vi "Sequence Module.vi"(0 "control_request":string, 5 "control_sequence_file_path":path, 9 "control_sequence_parameters":T3, 11 "control_sequence_current_parameters":T1) -> (3 "indicator_sequence_current_parameters":T1, 4 "indicator_sequence_parameters":T2, 6 "indicator_sequence_move_x":bool, 8 "indicator_UV_activation_intensity":dbl, 10 "indicator_sequence_move_y":bool, 13 "indicator_sequence_distance_y":dbl, 14 "indicator_UV_activation_time":dbl, 15 "indicator_sequence_distance_x":dbl)   [LabVIEW 2020]
uses:
  <vilib>/Utility/file.llb/Read Delimited Spreadsheet (string).vi
panel:
  out "indicator_saved_positions":i64[][](array[numeric])
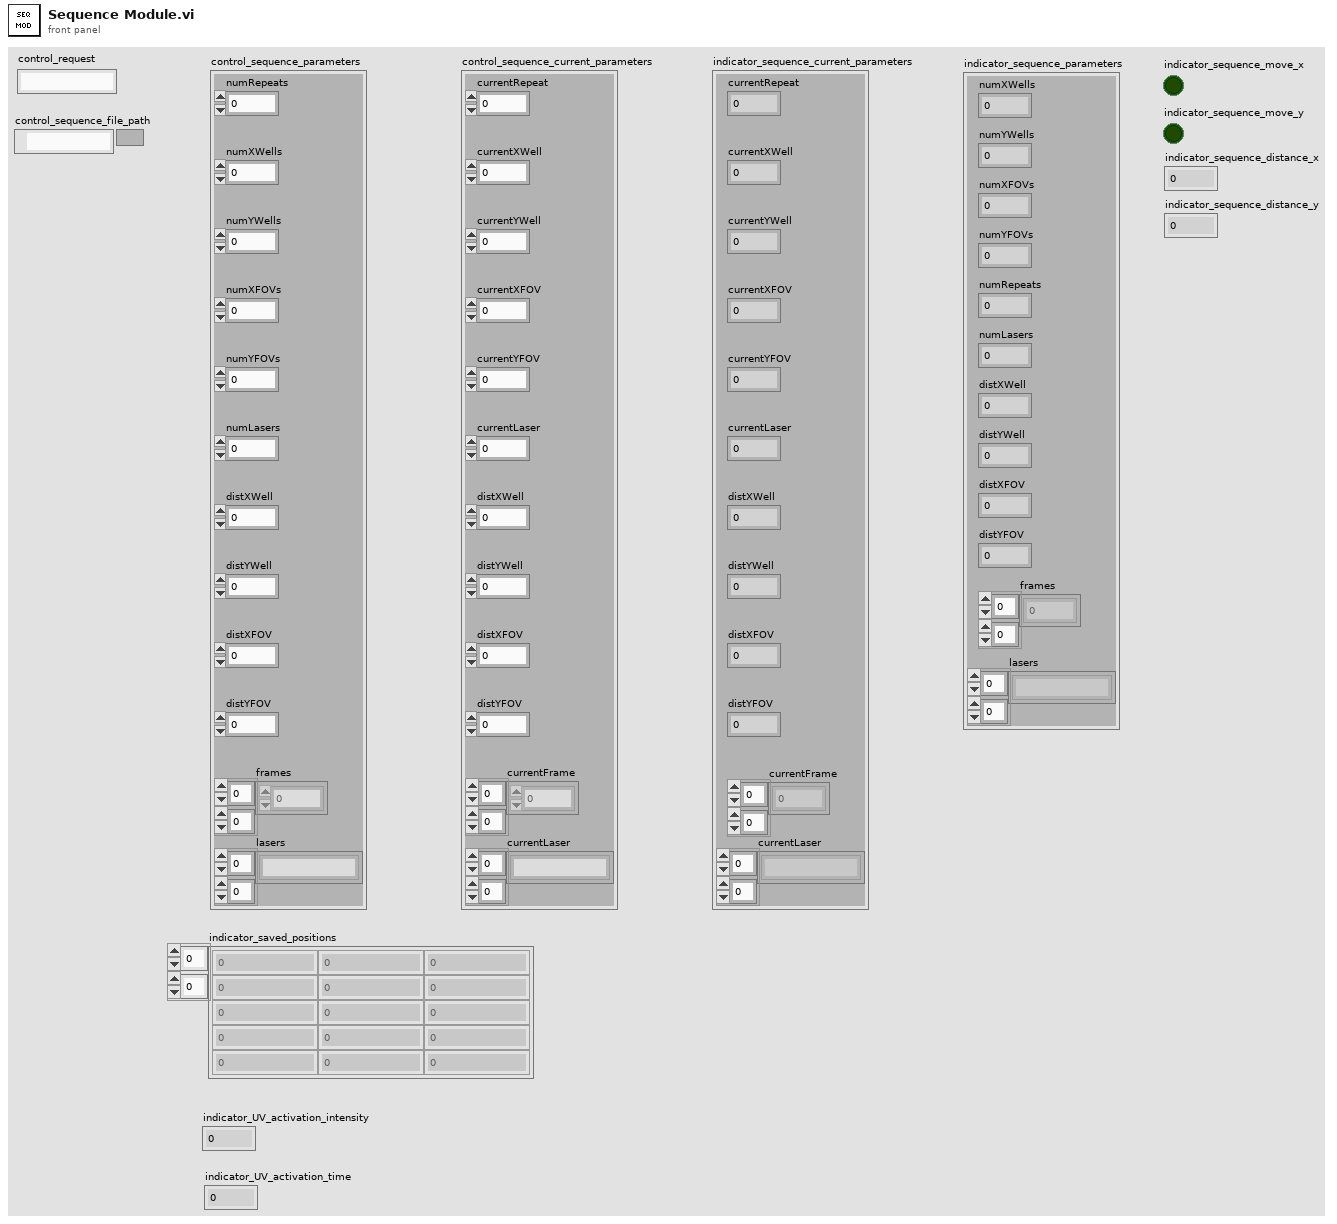
[diagram p1: front panel]
types:
  T1 = cluster{"currentXWell":i32, "currentYWell":i32, "currentXFOV":i32, "currentYFOV":i32, "currentRepeat":i32, "currentLaser":i32, "distXWell":i32, "distYWell":i32, "distXFOV":i32, "distYFOV":i32, "currentFrame":i32[][], "currentLaser":string[][]}
  T2 = cluster{"numXWells":i32, "numYWells":i32, "numXFOVs":i32, "numYFOVs":i32, "numRepeats":i32, "numLasers":i32, "distXWell":i32, "distYWell":i32, "distXFOV":i32, "distYFOV":i32, "frames":i32[][], "lasers":string[][]}
  T3 = cluster{"numXWells":i32, "numYWells":i32, "numXFOVs":i32, "numYFOVs":i32, "numRepeats":i32, "numLasers":i32, "distXWell":i32, "distYWell":i32, "distXFOV":i32, "distYFOV":i32, "frames":u32[][], "lasers":string[][]}
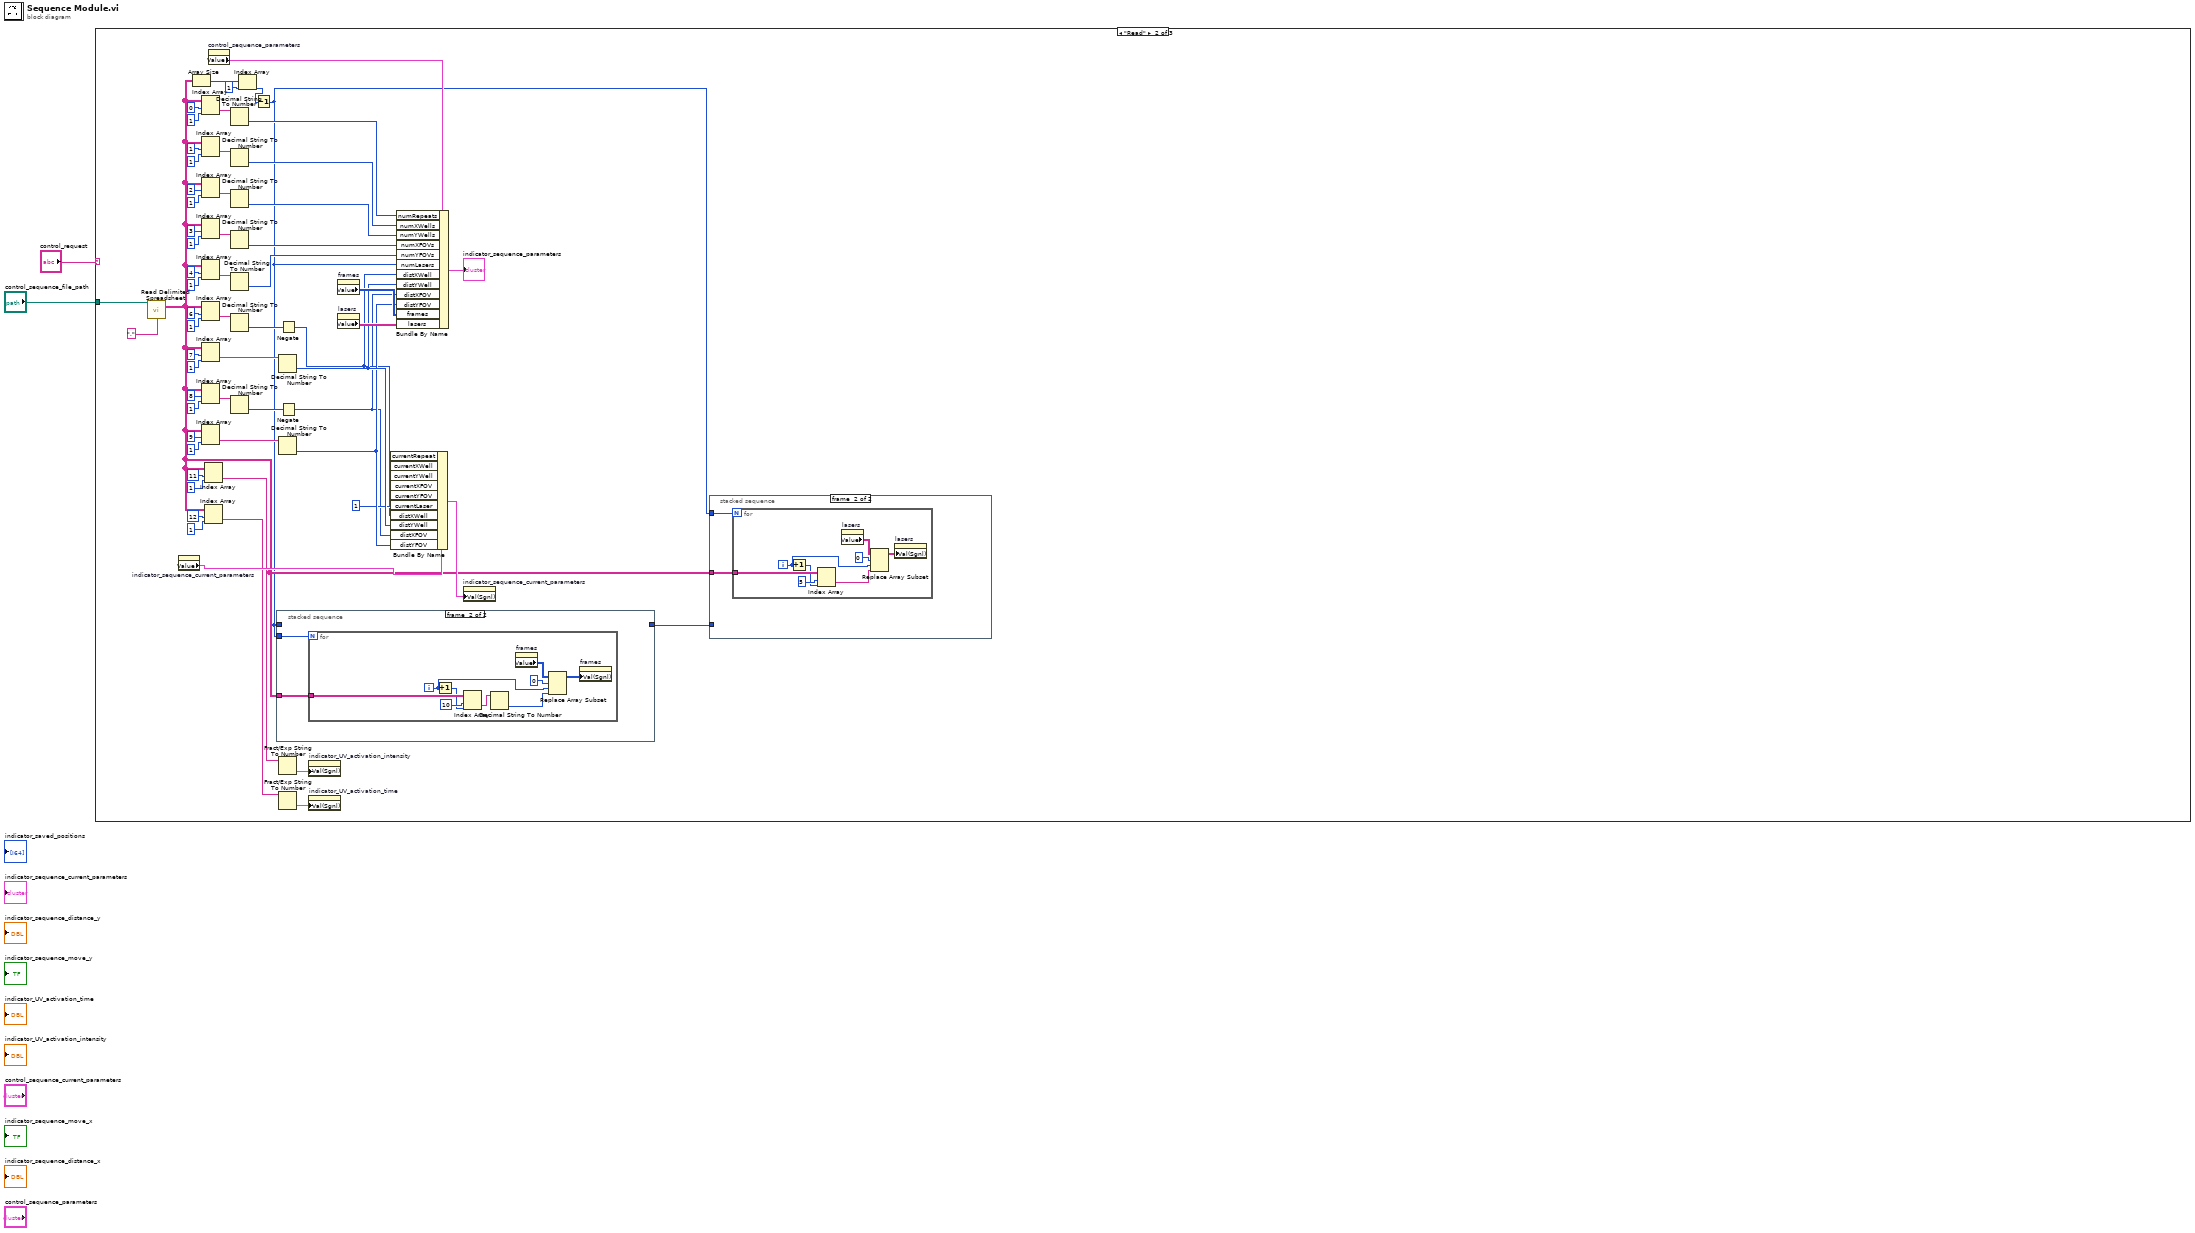
[diagram p0: block diagram]
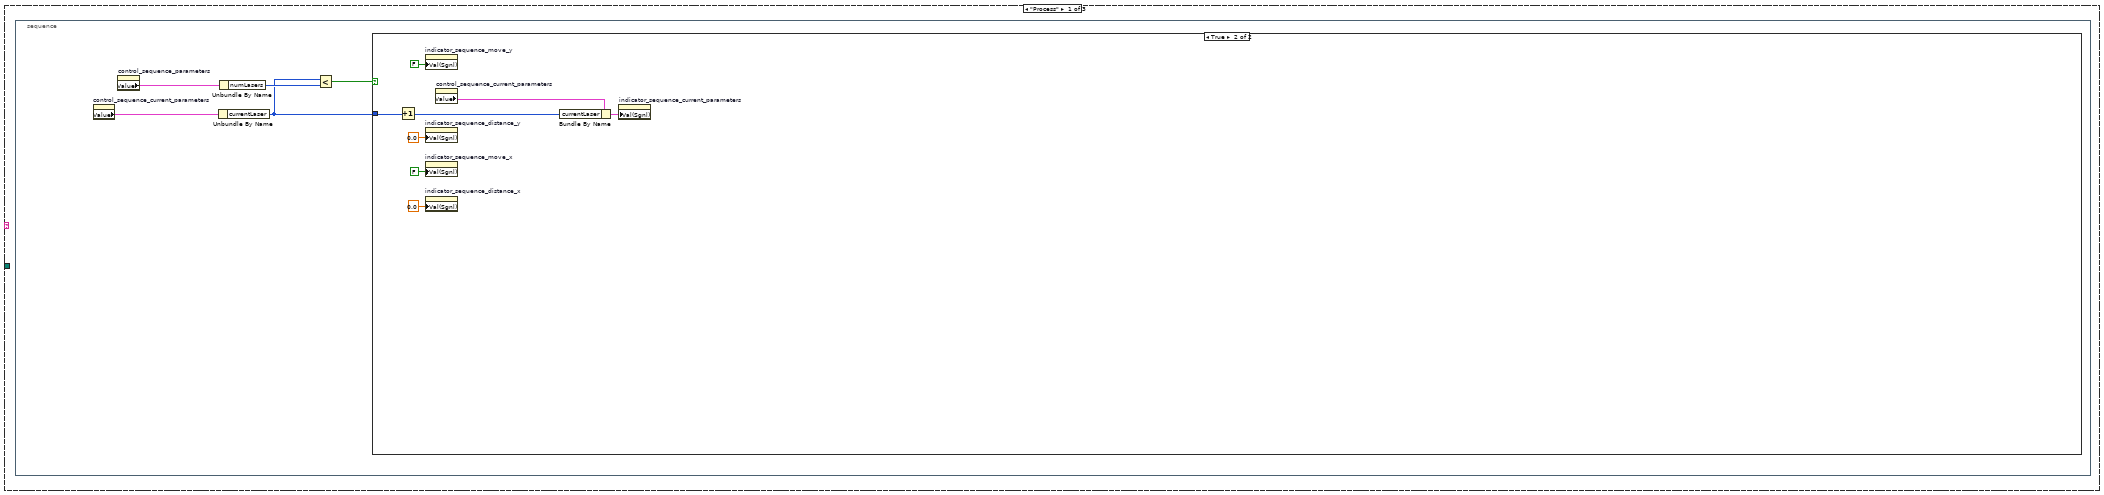
[diagram p2: hidden frame]
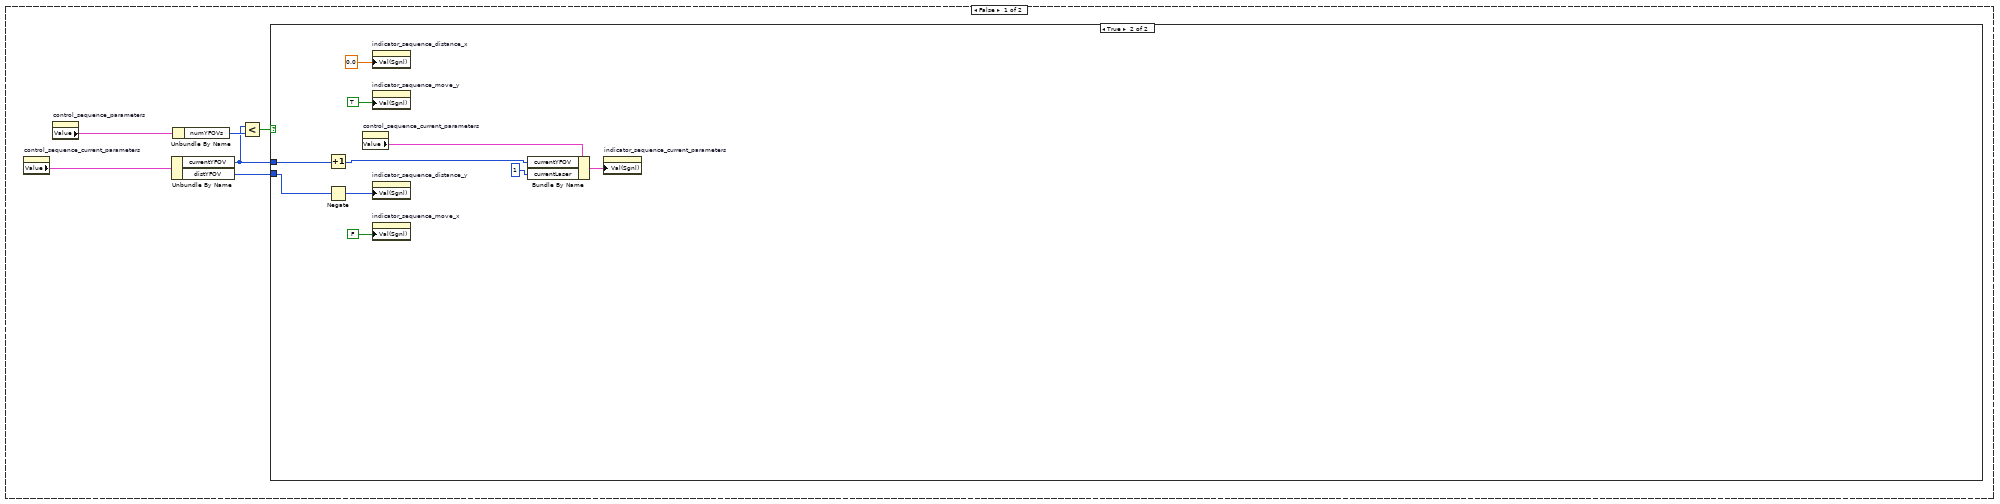
[diagram p3: hidden frame]
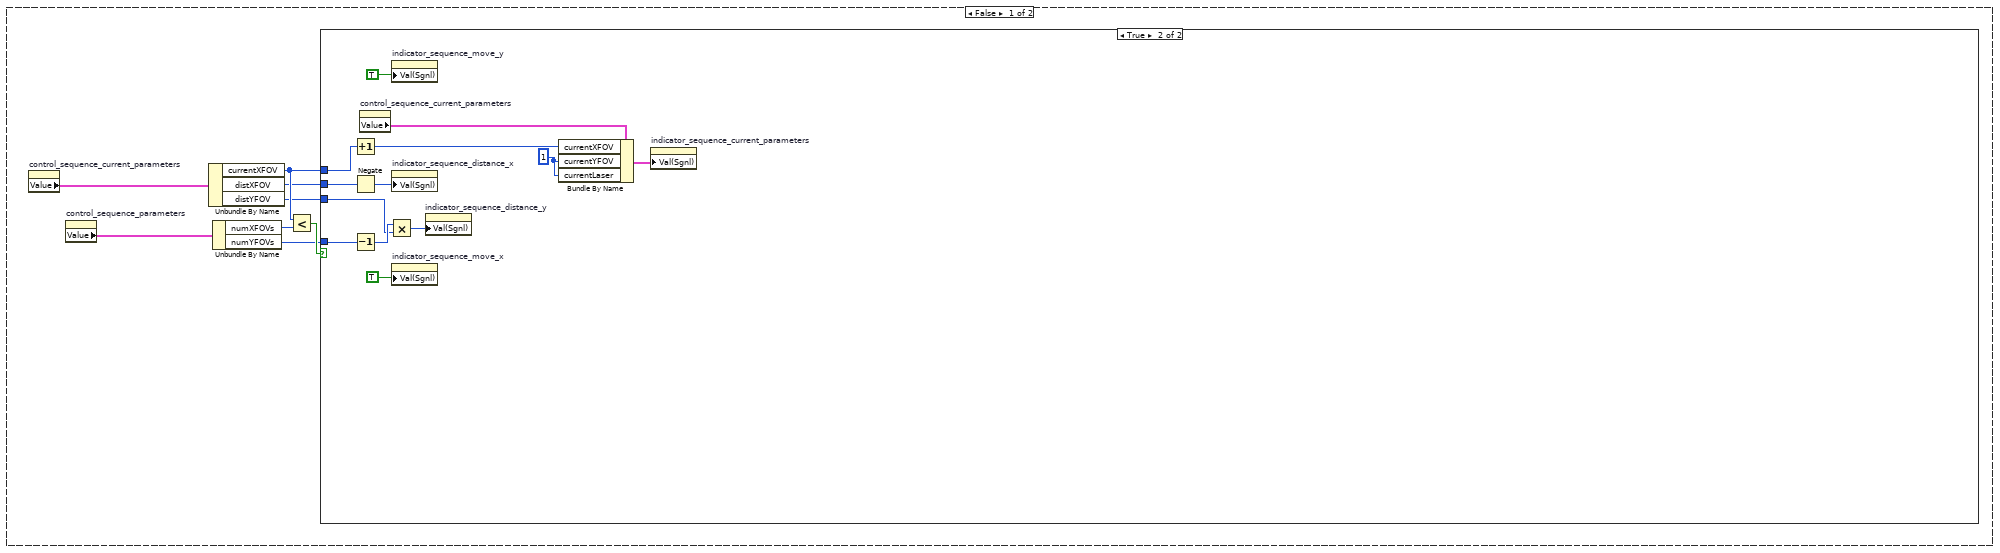
[diagram p4: hidden frame]
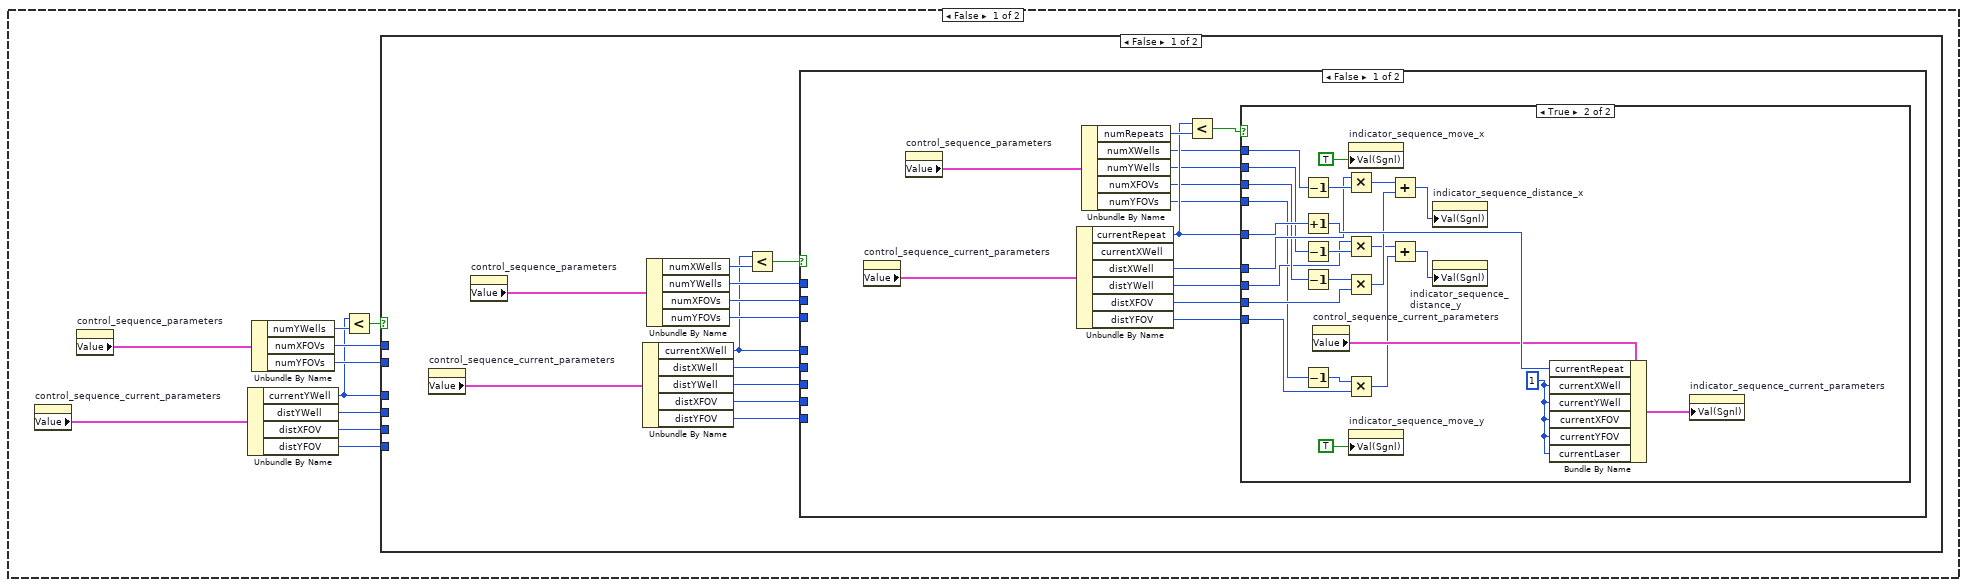
[diagram p5: hidden frame]
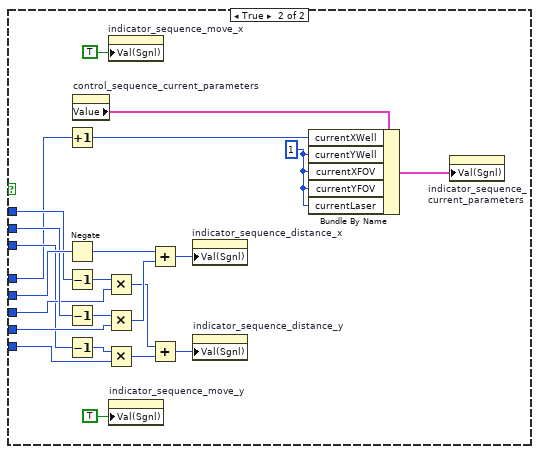
[diagram p7: hidden frame]
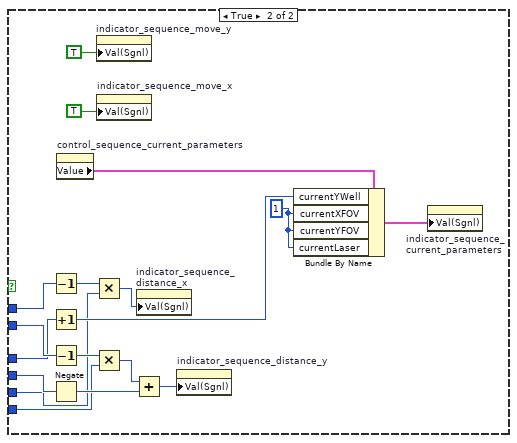
[diagram p8: hidden frame]
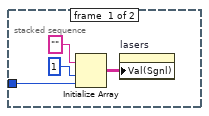
[diagram p9: hidden frame]
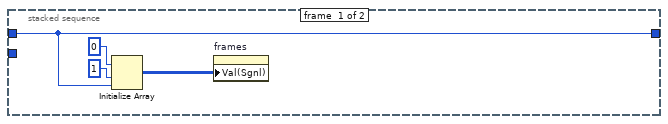
[diagram p10: hidden frame]
diagram:
  n1 = case shown="\"Read\"" "control_request" {
    tunnel: "control_sequence_file_path" -> [_ w171 _]
    frame "Process" {
      n2 = stacked-sequence {
        frame #0 {
          n3 = property on="control_sequence_current_parameters" class="Clust (strict)"() -> ("Value"=w6:T1)  [unwired: 2 in, 2 out]
          n4 = property on="control_sequence_parameters" class="Clust (strict)"() -> ("Value"=w5:T3)  [unwired: 2 in, 2 out]
          n5 = Unbundle By Name(w6) -> ("currentLaser"=w3:i32)
          n6 = Unbundle By Name(w5) -> ("numLasers"=w4:i32)
          n7 = Less?(x=w3, y=w4) -> (x < y?=w7:bool)
          n8 = case shown="True" w7 {
            tunnel: w3 -> [_ w146]
            frame False {
              n9 = property on="control_sequence_current_parameters" class="Clust (strict)"() -> ("Value"=w12:T1)  [unwired: 2 in, 2 out]
              n10 = property on="control_sequence_parameters" class="Clust (strict)"() -> ("Value"=w11:T3)  [unwired: 2 in, 2 out]
              n11 = Unbundle By Name(w12) -> ("currentYFOV"=w8:i32, "distYFOV"=w9:i32)
              n12 = Unbundle By Name(w11) -> ("numYFOVs"=w10:i32)
              n13 = Less?(x=w8, y=w10) -> (x < y?=w13:bool)
              n14 = case shown="True" w13 {
                tunnel: w9 -> [_ w137]
                tunnel: w8 -> [_ w136]
                frame False {
                  n15 = property on="control_sequence_current_parameters" class="Clust (strict)"() -> ("Value"=w20:T1)  [unwired: 2 in, 2 out]
                  n16 = property on="control_sequence_parameters" class="Clust (strict)"() -> ("Value"=w19:T3)  [unwired: 2 in, 2 out]
                  n17 = Unbundle By Name(w20) -> ("currentXFOV"=w17:i32, "distXFOV"=w16:i32, "distYFOV"=w14:i32)
                  n18 = Unbundle By Name(w19) -> ("numXFOVs"=w18:i32, "numYFOVs"=w15:i32)
                  n19 = Less?(x=w17, y=w18) -> (x < y?=w21:bool)
                  n20 = case shown="True" w21 {
                    tunnel: w17 -> [_ w126]
                    tunnel: w16 -> [_ w125]
                    tunnel: w15 -> [_ w124]
                    tunnel: w14 -> [_ w123]
                    frame False {
                      n21 = property on="control_sequence_current_parameters" class="Clust (strict)"() -> ("Value"=w30:T1)  [unwired: 2 in, 2 out]
                      n22 = property on="control_sequence_parameters" class="Clust (strict)"() -> ("Value"=w29:T3)  [unwired: 2 in, 2 out]
                      n23 = Unbundle By Name(w30) -> ("currentYWell"=w22:i32, "distYWell"=w27:i32, "distXFOV"=w23:i32, "distYFOV"=w25:i32)
                      n24 = Unbundle By Name(w29) -> ("numYWells"=w28:i32, "numXFOVs"=w24:i32, "numYFOVs"=w26:i32)
                      n25 = Less?(x=w22, y=w28) -> (x < y?=w31:bool)
                      n26 = case shown="False" w31 {
                        tunnel: w27 -> [_ w110]
                        tunnel: w26 -> [_ w109]
                        tunnel: w25 -> [_ w108]
                        tunnel: w24 -> [_ w107]
                        tunnel: w23 -> [_ w106]
                        tunnel: w22 -> [_ w105]
                        frame False {
                          n27 = property on="control_sequence_current_parameters" class="Clust (strict)"() -> ("Value"=w42:T1)  [unwired: 2 in, 2 out]
                          n28 = property on="control_sequence_parameters" class="Clust (strict)"() -> ("Value"=w41:T3)  [unwired: 2 in, 2 out]
                          n29 = Unbundle By Name(w42) -> ("currentXWell"=w32:i32, "distXWell"=w39:i32, "distYWell"=w35:i32, "distXFOV"=w37:i32, "distYFOV"=w33:i32)
                          n30 = Unbundle By Name(w41) -> ("numXWells"=w40:i32, "numYWells"=w36:i32, "numXFOVs"=w38:i32, "numYFOVs"=w34:i32)
                          n31 = Less?(x=w32, y=w40) -> (x < y?=w43:bool)
                          n32 = case shown="False" w43 {
                            tunnel: w39 -> [_ w89]
                            tunnel: w38 -> [_ w88]
                            tunnel: w37 -> [_ w87]
                            tunnel: w36 -> [_ w86]
                            tunnel: w35 -> [_ w85]
                            tunnel: w34 -> [_ w84]
                            tunnel: w33 -> [_ w83]
                            tunnel: w32 -> [_ w82]
                            frame False {
                              n33 = property on="control_sequence_current_parameters" class="Clust (strict)"() -> ("Value"=w55:T1)  [unwired: 2 in, 2 out]
                              n34 = property on="control_sequence_parameters" class="Clust (strict)"() -> ("Value"=w54:T3)  [unwired: 2 in, 2 out]
                              n35 = Unbundle By Name(w55) -> ("currentRepeat"=w52:i32, "distXWell"=w50:i32, "distYWell"=w47:i32, "distXFOV"=w48:i32, "distYFOV"=w45:i32)  [unwired: 1 out]
                              n36 = Unbundle By Name(w54) -> ("numRepeats"=w53:i32, "numXWells"=w51:i32, "numYWells"=w46:i32, "numXFOVs"=w49:i32, "numYFOVs"=w44:i32)
                              n37 = Less?(x=w52, y=w53) -> (x < y?=w56:bool)
                              n38 = case shown="True" w56 {
                                tunnel: w52 -> [_ w75]
                                tunnel: w51 -> [_ w74]
                                tunnel: w50 -> [_ w72]
                                tunnel: w49 -> [_ w68]
                                tunnel: w48 -> [_ w67]
                                tunnel: w47 -> [_ w60]
                                tunnel: w46 -> [_ w59]
                                tunnel: w45 -> [_ w58]
                                tunnel: w44 -> [_ w57]
                                frame False {
                                }
                                frame True {
                                w78 = 1 ("currentXWell")
                                n39 = Decrement(x=w74) -> (x-1=w73:i32)
                                n40 = Increment(x=w75) -> (x+1=w80:i32)
                                n41 = Decrement(x=w59) -> (x-1=w65:i32)
                                n42 = Decrement(x=w68) -> (x-1=w69:i32)
                                n43 = Decrement(x=w57) -> (x-1=w62:i32)
                                n44 = property on="control_sequence_current_parameters" class="Clust (strict)"() -> ("Value"=w79:T1)  [unwired: 2 in, 2 out]
                                n45 = Multiply(x=w72, y=w73) -> (x*y=w71:i32)
                                n46 = Multiply(x=w60, y=w65) -> (x*y=w64:i32)
                                n47 = Multiply(x=w69, y=w67) -> (x*y=w70:i32)
                                n48 = Multiply(x=w62, y=w58) -> (x*y=w63:i32)
                                n49 = property on="indicator_sequence_move_x" class="Bool (strict)"("Val(Sgnl)"=TRUE ("Value (Signaling)")) -> ()  [unwired: 2 in, 2 out]
                                n50 = property on="indicator_sequence_move_y" class="Bool (strict)"("Val(Sgnl)"=TRUE ("Value (Signaling)")) -> ()  [unwired: 2 in, 2 out]
                                n51 = Add(x=w71, y=w70) -> (x+y=w66:i32)
                                n52 = Add(x=w64, y=w63) -> (x+y=w61:i32)
                                n53 = property on="indicator_sequence_distance_x" class="DigNum (strict)"("Val(Sgnl)"=w66) -> ()  [unwired: 2 in, 2 out]
                                n54 = property on="indicator_sequence_distance_y" class="DigNum (strict)"("Val(Sgnl)"=w61) -> ()  [unwired: 2 in, 2 out]
                                n55 = Bundle By Name(cluster=w79, "currentRepeat"=w80, "currentXWell"=w78, "currentYWell"=w78, "currentXFOV"=w78, "currentYFOV"=w78, "currentLaser"=w78) -> (w81:T1)
                                n56 = property on="indicator_sequence_current_parameters" class="Clust (strict)"("Val(Sgnl)"=w81) -> ()  [unwired: 2 in, 2 out]
                                }
                              }
                            }
                            frame True {
                              w101 = 1 ("currentYWell")
                              n57 = Increment(x=w82) -> (x+1=w103:i32)
                              n58 = Negate(x=w89) -> (-x=w95:i32)
                              n59 = Decrement(x=w86) -> (x-1=w98:i32)
                              n60 = Decrement(x=w88) -> (x-1=w97:i32)
                              n61 = Decrement(x=w84) -> (x-1=w96:i32)
                              n62 = property on="control_sequence_current_parameters" class="Clust (strict)"() -> ("Value"=w102:T1)  [unwired: 2 in, 2 out]
                              n63 = Multiply(x=w98, y=w85) -> (x*y=w92:i32)
                              n64 = Multiply(x=w97, y=w87) -> (x*y=w94:i32)
                              n65 = Multiply(x=w96, y=w83) -> (x*y=w91:i32)
                              n66 = property on="indicator_sequence_move_x" class="Bool (strict)"("Val(Sgnl)"=TRUE ("Value (Signaling)")) -> ()  [unwired: 2 in, 2 out]
                              n67 = property on="indicator_sequence_move_y" class="Bool (strict)"("Val(Sgnl)"=TRUE ("Value (Signaling)")) -> ()  [unwired: 2 in, 2 out]
                              n68 = Add(x=w95, y=w94) -> (x+y=w93:i32)
                              n69 = Add(x=w92, y=w91) -> (x+y=w90:i32)
                              n70 = property on="indicator_sequence_distance_x" class="DigNum (strict)"("Val(Sgnl)"=w93) -> ()  [unwired: 2 in, 2 out]
                              n71 = property on="indicator_sequence_distance_y" class="DigNum (strict)"("Val(Sgnl)"=w90) -> ()  [unwired: 2 in, 2 out]
                              n72 = Bundle By Name(cluster=w102, "currentXWell"=w103, "currentYWell"=w101, "currentXFOV"=w101, "currentYFOV"=w101, "currentLaser"=w101) -> (w104:T1)
                              n73 = property on="indicator_sequence_current_parameters" class="Clust (strict)"("Val(Sgnl)"=w104) -> ()  [unwired: 2 in, 2 out]
                            }
                          }
                        }
                        frame True {
                          w119 = 1 ("currentXFOV")
                          n74 = Decrement(x=w107) -> (x-1=w116:i32)
                          n75 = Increment(x=w105) -> (x+1=w121:i32)
                          n76 = Decrement(x=w109) -> (x-1=w114:i32)
                          n77 = Negate(x=w110) -> (-x=w113:i32)
                          n78 = property on="control_sequence_current_parameters" class="Clust (strict)"() -> ("Value"=w120:T1)  [unwired: 2 in, 2 out]
                          n79 = Multiply(x=w116, y=w106) -> (x*y=w115:i32)
                          n80 = Multiply(x=w114, y=w108) -> (x*y=w112:i32)
                          n81 = property on="indicator_sequence_move_y" class="Bool (strict)"("Val(Sgnl)"=TRUE ("Value (Signaling)")) -> ()  [unwired: 2 in, 2 out]
                          n82 = property on="indicator_sequence_move_x" class="Bool (strict)"("Val(Sgnl)"=TRUE ("Value (Signaling)")) -> ()  [unwired: 2 in, 2 out]
                          n83 = Add(x=w112, y=w113) -> (x+y=w111:i32)
                          n84 = property on="indicator_sequence_distance_x" class="DigNum (strict)"("Val(Sgnl)"=w115) -> ()  [unwired: 2 in, 2 out]
                          n85 = property on="indicator_sequence_distance_y" class="DigNum (strict)"("Val(Sgnl)"=w111) -> ()  [unwired: 2 in, 2 out]
                          n86 = Bundle By Name(cluster=w120, "currentYWell"=w121, "currentXFOV"=w119, "currentYFOV"=w119, "currentLaser"=w119) -> (w122:T1)
                          n87 = property on="indicator_sequence_current_parameters" class="Clust (strict)"("Val(Sgnl)"=w122) -> ()  [unwired: 2 in, 2 out]
                        }
                      }
                    }
                    frame True {
                      w132 = 1 ("currentYFOV")
                      n88 = Increment(x=w126) -> (x+1=w135:i32)
                      n89 = Negate(x=w125) -> (-x=w129:i32)
                      n90 = Decrement(x=w124) -> (x-1=w128:i32)
                      n91 = property on="control_sequence_current_parameters" class="Clust (strict)"() -> ("Value"=w133:T1)  [unwired: 2 in, 2 out]
                      n92 = Multiply(x=w128, y=w123) -> (x*y=w127:i32)
                      n93 = property on="indicator_sequence_move_y" class="Bool (strict)"("Val(Sgnl)"=TRUE ("Value (Signaling)")) -> ()  [unwired: 2 in, 2 out]
                      n94 = property on="indicator_sequence_distance_x" class="DigNum (strict)"("Val(Sgnl)"=w129) -> ()  [unwired: 2 in, 2 out]
                      n95 = property on="indicator_sequence_move_x" class="Bool (strict)"("Val(Sgnl)"=TRUE ("Value (Signaling)")) -> ()  [unwired: 2 in, 2 out]
                      n96 = property on="indicator_sequence_distance_y" class="DigNum (strict)"("Val(Sgnl)"=w127) -> ()  [unwired: 2 in, 2 out]
                      n97 = Bundle By Name(cluster=w133, "currentXFOV"=w135, "currentYFOV"=w132, "currentLaser"=w132) -> (w134:T1)
                      n98 = property on="indicator_sequence_current_parameters" class="Clust (strict)"("Val(Sgnl)"=w134) -> ()  [unwired: 2 in, 2 out]
                    }
                  }
                }
                frame True {
                  n99 = Increment(x=w136) -> (x+1=w143:i32)
                  n100 = Negate(x=w137) -> (-x=w139:i32)
                  n101 = property on="control_sequence_current_parameters" class="Clust (strict)"() -> ("Value"=w144:T1)  [unwired: 2 in, 2 out]
                  n102 = property on="indicator_sequence_distance_x" class="DigNum (strict)"("Val(Sgnl)"=0.0 ("Value (Signaling)")) -> ()  [unwired: 2 in, 2 out]
                  n103 = property on="indicator_sequence_move_y" class="Bool (strict)"("Val(Sgnl)"=TRUE ("Value (Signaling)")) -> ()  [unwired: 2 in, 2 out]
                  n104 = property on="indicator_sequence_distance_y" class="DigNum (strict)"("Val(Sgnl)"=w139) -> ()  [unwired: 2 in, 2 out]
                  n105 = property on="indicator_sequence_move_x" class="Bool (strict)"("Val(Sgnl)"=FALSE ("Value (Signaling)")) -> ()  [unwired: 2 in, 2 out]
                  n106 = Bundle By Name(cluster=w144, "currentYFOV"=w143, "currentLaser"=1) -> (w145:T1)
                  n107 = property on="indicator_sequence_current_parameters" class="Clust (strict)"("Val(Sgnl)"=w145) -> ()  [unwired: 2 in, 2 out]
                }
              }
            }
            frame True {
              n108 = Increment(x=w146) -> (x+1=w153:i32)
              n109 = property on="indicator_sequence_move_y" class="Bool (strict)"("Val(Sgnl)"=FALSE ("Value (Signaling)")) -> ()  [unwired: 2 in, 2 out]
              n110 = property on="indicator_sequence_distance_y" class="DigNum (strict)"("Val(Sgnl)"=0.0 ("Value (Signaling)")) -> ()  [unwired: 2 in, 2 out]
              n111 = property on="indicator_sequence_move_x" class="Bool (strict)"("Val(Sgnl)"=FALSE ("Value (Signaling)")) -> ()  [unwired: 2 in, 2 out]
              n112 = property on="indicator_sequence_distance_x" class="DigNum (strict)"("Val(Sgnl)"=0.0 ("Value (Signaling)")) -> ()  [unwired: 2 in, 2 out]
              n113 = property on="control_sequence_current_parameters" class="Clust (strict)"() -> ("Value"=w151:T1)  [unwired: 2 in, 2 out]
              n114 = Bundle By Name(cluster=w151, "currentLaser"=w153) -> (w152:T1)
              n115 = property on="indicator_sequence_current_parameters" class="Clust (strict)"("Val(Sgnl)"=w152) -> ()  [unwired: 2 in, 2 out]
            }
          }
        }
      }
    }
    frame "Read" {
      w170 = 1 ("currentLaser")
      n116 = call-poly <vilib>:"Read Delimited Spreadsheet.vi"("file path (dialog if empty)"=w171, "delimiter (\\t)"="," ("delimiter (\\t)")) -> ("all rows"=w157:string[][])  [unwired: 8 in, 5 out]
      n117 = property on="indicator_sequence_current_parameters" class="Clust (strict)"() -> ("Value"=w179:T1)  [unwired: 2 in, 2 out]
      n118 = Array Size(array=w157) -> (size(s)=w189:i32[])
      n119 = Index Array(array=w157, index (row)=0 ("index"), index (col)=1 ("disabled index (col)")) -> (element=w195:string)
      n120 = Index Array(array=w157, index (row)=1 ("index"), index (col)=1 ("disabled index (col)")) -> (element=w194:string)
      n121 = Index Array(array=w157, index (row)=2 ("index"), index (col)=1 ("disabled index (col)")) -> (element=w193:string)
      n122 = Index Array(array=w157, index (row)=3 ("index"), index (col)=1 ("disabled index (col)")) -> (element=w192:string)
      n123 = Index Array(array=w157, index (row)=4 ("index"), index (col)=1 ("disabled index (col)")) -> (element=w191:string)
      n124 = Index Array(array=w157, index (row)=6 ("index"), index (col)=1 ("disabled index (col)")) -> (element=w188:string)
      n125 = Index Array(array=w157, index (row)=7 ("index"), index (col)=1 ("disabled index (col)")) -> (element=w187:string)
      n126 = Index Array(array=w157, index (row)=8 ("index"), index (col)=1 ("disabled index (col)")) -> (element=w186:string)
      n127 = Index Array(array=w157, index (row)=9 ("index"), index (col)=1 ("disabled index (col)")) -> (element=w185:string)
      n128 = Index Array(array=w157, index (row)=11, index (col)=1 ("disabled index (col)")) -> (element=w162:string)
      n129 = Index Array(array=w157, index (row)=12, index (col)=1 ("disabled index (col)")) -> (element=w158:string)
      n130 = property on="control_sequence_parameters" class="Clust (strict)"() -> ("Value"=w169:T3)  [unwired: 2 in, 2 out]
      n131 = Decimal String To Number(string=w195) -> (number=w178:i32)  [unwired: 2 in, 1 out]
      n132 = Decimal String To Number(string=w194) -> (number=w177:i32)  [unwired: 2 in, 1 out]
      n133 = Decimal String To Number(string=w193) -> (number=w176:i32)  [unwired: 2 in, 1 out]
      n134 = Decimal String To Number(string=w192) -> (number=w175:i32)  [unwired: 2 in, 1 out]
      n135 = Decimal String To Number(string=w191) -> (number=w174:i32)  [unwired: 2 in, 1 out]
      n136 = Decimal String To Number(string=w188) -> (number=w168:i32)  [unwired: 2 in, 1 out]
      n137 = Decimal String To Number(string=w186) -> (number=w166:i32)  [unwired: 2 in, 1 out]
      n138 = Index Array(array=w189, index=1) -> (element=w155:i32)
      n139 = Decrement(x=w155) -> (x-1=w154:i32)
      n140 = stacked-sequence {
        tunnel: w154 -> [w230 _]
        tunnel: [w230 _] -> w184
        tunnel: w154 -> [_ w234]
        tunnel: w157 -> [_ w233]
        frame #0 {
          n141 = Initialize Array(0 ("element"), 1 ("dimension size"), w230) -> (w229:i32[][])
          n142 = property on="frames" class="Arr (strict)"("Val(Sgnl)"=w229) -> ()  [unwired: 2 in, 2 out]
        }
        frame #1 {
          n143 = for {
            N: w234 -> [_]
            tunnel: w233 -> [w243]
            i -> [w235]
            n144 = Increment(x=w235) -> (x+1=w236:i32)
            n145 = Index Array(array=w243, index (row)=10 ("index"), index (col)=w236) -> (element=w241:string)
            n146 = Decimal String To Number(string=w241) -> (number=w239:i32)  [unwired: 2 in, 1 out]
            n147 = property on="frames" class="Arr (strict)"() -> ("Value"=w237:i32[][])  [unwired: 2 in, 2 out]
            n148 = Replace Array Subset(array=w237, new element=w239, index (row)=0, index (col)=w235) -> (w238:i32[][])
            n149 = property on="frames" class="Arr (strict)"("Val(Sgnl)"=w238) -> ()  [unwired: 2 in, 2 out]
          }
        }
      }
      n150 = Decimal String To Number(string=w187) -> (number=w173:i32)  [unwired: 2 in, 1 out]
      n151 = Decimal String To Number(string=w185) -> (number=w172:i32)  [unwired: 2 in, 1 out]
      n152 = Fract/Exp String To Number(string=w162) -> (number=w161:dbl)  [unwired: 3 in, 1 out]
      n153 = Fract/Exp String To Number(string=w158) -> (number=w156:dbl)  [unwired: 3 in, 1 out]
      n154 = Negate(x=w168) -> (-x=w167:i32)
      n155 = Negate(x=w166) -> (-x=w165:i32)
      n156 = property on="indicator_UV_activation_intensity" class="DigNum (strict)"("Val(Sgnl)"=w161) -> ()  [unwired: 2 in, 2 out]
      n157 = property on="indicator_UV_activation_time" class="DigNum (strict)"("Val(Sgnl)"=w156) -> ()  [unwired: 2 in, 2 out]
      n158 = property on="frames" class="Arr (strict)"() -> ("Value"=w182:i32[][])  [unwired: 2 in, 2 out]
      n159 = property on="lasers" class="Arr (strict)"() -> ("Value"=w181:string[][])  [unwired: 2 in, 2 out]
      n160 = Bundle By Name(cluster=w179, "currentRepeat"=w170, "currentXWell"=w170, "currentYWell"=w170, "currentXFOV"=w170, "currentYFOV"=w170, "currentLaser"=w170, "distXWell"=w167, "distYWell"=w173, "distXFOV"=w165, "distYFOV"=w172) -> (w180:T1)
      n161 = Bundle By Name(cluster=w169, "numRepeats"=w178, "numXWells"=w177, "numYWells"=w176, "numXFOVs"=w175, "numYFOVs"=w174, "numLasers"=w154, "distXWell"=w167, "distYWell"=w173, "distXFOV"=w165, "distYFOV"=w172, "frames"=w182, "lasers"=w181) -> (→"indicator_sequence_parameters":T3)
      n162 = property on="indicator_sequence_current_parameters" class="Clust (strict)"("Val(Sgnl)"=w180) -> ()  [unwired: 2 in, 2 out]
      n163 = stacked-sequence {
        tunnel: w184 -> [w217 _]
        tunnel: w154 -> [_ w220]
        tunnel: w157 -> [_ w219]
        frame #0 {
          n164 = Initialize Array("", 1 ("dimension size"), w217) -> (w215:string[][])
          n165 = property on="lasers" class="Arr (strict)"("Val(Sgnl)"=w215) -> ()  [unwired: 2 in, 2 out]
        }
        frame #1 {
          n166 = for {
            N: w220 -> [_]
            tunnel: w219 -> [w228]
            i -> [w221]
            n167 = Increment(x=w221) -> (x+1=w222:i32)
            n168 = Index Array(array=w228, index (row)=5 ("index"), index (col)=w222) -> (element=w225:string)
            n169 = property on="lasers" class="Arr (strict)"() -> ("Value"=w223:string[][])  [unwired: 2 in, 2 out]
            n170 = Replace Array Subset(array=w223, new element=w225, index (row)=0, index (col)=w221) -> (w224:string[][])
            n171 = property on="lasers" class="Arr (strict)"("Val(Sgnl)"=w224) -> ()  [unwired: 2 in, 2 out]
          }
        }
      }
    }
    frame "Default", Default {
    }
  }
